vi "Modelo.vi"() -> ()   [LabVIEW 2016]
uses:
  <vilib>/addons/System Identification/Model Typedefs.llb/si_generic model.ctl
  <vilib>/addons/System Identification/Model Typedefs.llb/SI Model Type.ctl
  <vilib>/addons/System Identification/Model Typedefs.llb/si_variables.ctl
  <vilib>/addons/Control Design/_Model Construction/Model Typedefs.llb/CD Transfer Function Model (MIMO).ctl
  <vilib>/addons/Control Design/_Model Construction/Model Typedefs.llb/CD General Elements.ctl
  <vilib>/addons/Control Design/_Model Construction/Model Typedefs.llb/CD Transfer Function Model (SISO).ctl
  <vilib>/addons/Control Design/_PID Design/Datatypes/cd_PID Gains.ctl
  <vilib>/addons/Control Design/_PID Design/Datatypes/cd_Sampling Specifications.ctl
  <vilib>/Utility/file.llb/Read Delimited Spreadsheet (DBL).vi
  <vilib>/addons/Control Design/_Model Construction/Model Creation.llb/Model Creation SubVI/cd_Create Transfer Function Model.vi
  <vilib>/addons/Control Design/_PID Design/cd_Design PID for Discrete Systems (TF).vi
  <vilib>/Analysis/NI_AALPro.lvlib
  <vilib>/addons/Control Design/_PID Design/NI_CD_PID Design.lvlib
  <vilib>/addons/Control Design/_Model Construction/NI_LinSys_Model Creation.lvlib
  <vilib>/addons/System Identification/NI_SysID.lvlib
  <vilib>/addons/Control Design/_Model Construction/NI_LinSys_Model Typedefs.lvlib
panel:
  out "Design PID Gains":T1
  out "output cluster":T2 {"transfer function(s)"."delay" format="%.4f"; "transfer function(s)"."Denominator" format="%#_3g"; "transfer function(s)"."Numerator" format="%#_3g"; "properties"."Sampling Time" format="%#.6p"; "properties"."Output Delays" format="%.4f"; "properties"."Input Delays" format="%.4f"}
  out "size(s)":i32
  out "Waveform Graph":dbl[](graph)
  in  "file path (dialog if empty)":path
  out "coefficients":cluster{"numerator":dbl[], "denominator":dbl[]}
  out "system model out":T5={"attributes"={"version"="1.0", "model type"=0, "input names"=[], "output names"=[], "notes"=""}, "coefficients"={"A "=[], "B"=[], "F"=[], "C"=[], "D"=[]}, "std deviations"={"A "=[], "B"=[], "F"=[], "C"=[], "D"=[]}, "coefficients covariance"=[], "noise variance"=[], "fs"=0.0, "system info"={"number of inputs"=0, "number of outputs"=0, "A order"=[], "B order"=[], "F order"=[], "C order"=[], "D order"=[], "Delays"=[]}, "kalman gain"=[], "initial state"=[], "trans func"=[], "zeros-poles"=[], "std of trans func"=[], "std of zeros-poles"=[], "trans func (noise)"=[], "std of trans func (noise)"=[], "zeros-poles (noise)"=[], "std of zeros-poles (noise)"=[], "Symbolic State Space Model"={"Symbolic A"=[], "Symbolic B"=[], "Symbolic C"=[], "Symbolic D"=[], "Symbolic K"=[], "Symbolic Initial State"=[]}, "delay"=[], "variables"=[], "grey trans func spec"={"orders of TF model"={" num order"=1, "den order"=2}, "# of zeros/poles at origin"={"zeros/poles"=1, "number "=0}, "delay initial?"=FALSE, "gain initial?"=FALSE}} {"grey trans func spec"."# of zeros/poles at origin"."zeros/poles" items=["zeros", "poles"]; "std of zeros-poles (noise)"."gain" format="%.2f"; "std of zeros-poles (noise)"."poles" format="%.2f"; "std of zeros-poles (noise)"."zeros" format="%.2f"; "zeros-poles (noise)"."gain" format="%.2f"; "zeros-poles (noise)"."poles" format="%.2f"; "zeros-poles (noise)"."zeros" format="%.2f"; "std of trans func (noise)"."alphas" format="%.2f"; "std of trans func (noise)"."betas" format="%.2f"; "trans func (noise)"."alphas" format="%.2f"; "trans func (noise)"."betas" format="%.2f"; "std of zeros-poles"."gain" format="%.2f"; "std of zeros-poles"."poles" format="%.2f"; "std of zeros-poles"."zeros" format="%.2f"; "std of trans func"."alphas" format="%.2f"; "std of trans func"."betas" format="%.2f"; "zeros-poles"."gain" format="%.2f"; "zeros-poles"."poles" format="%.2f"; "zeros-poles"."zeros" format="%.2f"; "trans func"."alphas" format="%.2f"; "trans func"."betas" format="%.2f"; "fs" format="%.2f"; "std deviations"."A" format="%.2f"; "std deviations"."D" format="%.2f"; "std deviations"."C" format="%.2f"; "std deviations"."F" format="%.2f"; "std deviations"."B" format="%.2f"; "coefficients"."A" format="%.2f"; "coefficients"."D" format="%.2f"; "coefficients"."C" format="%.2f"; "coefficients"."F" format="%.2f"; "coefficients"."B" format="%.2f"; "attributes"."model type" items=["Undefined", "AR", "ARX (SISO)", "ARX (MISO)", "ARX (MIMO)", "ARMAX (SISO)", "ARMAX (MISO)", "Output-Error (SISO)", "Output-Error (MISO)", "Box-Jenkins (SISO)", "Box-Jenkins (MISO)", "General Linear (SISO)", "General Linear (MISO)", "State-Space (SISO)", "State-Space (MISO)", "State-Space (MIMO)", "Transfer Function (SISO)", "Transfer Function (MISO)", "Transfer Function (MIMO)", "Zero-Pole-Gain (SISO)", "Zero-Pole-Gain (MISO)", "Zero-Pole-Gain (MIMO)"]}
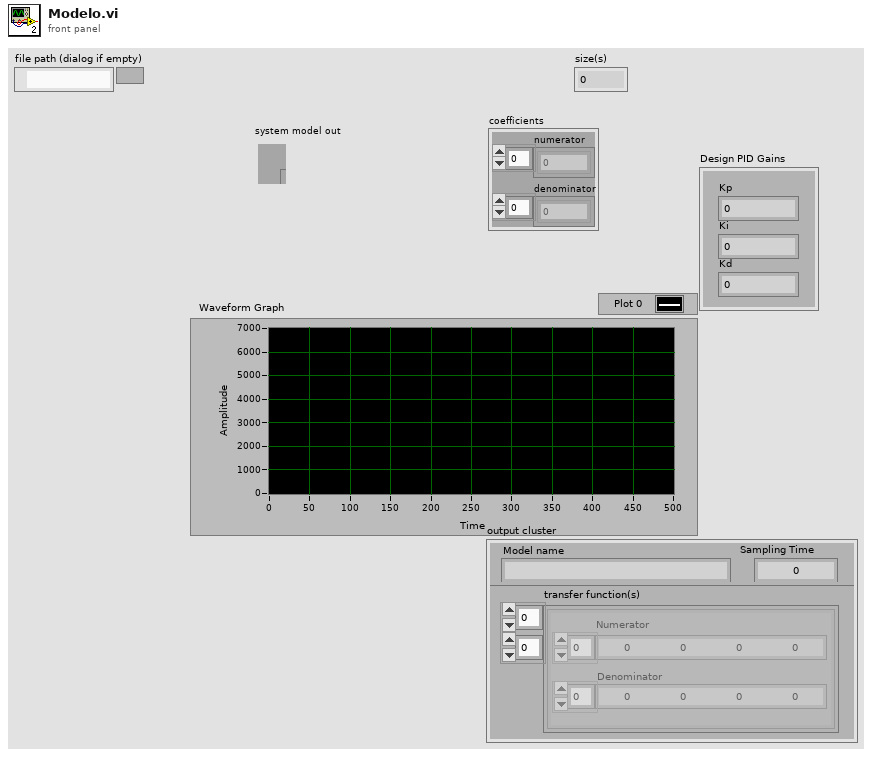
[diagram p1: front panel]
types:
  T1 = typedef "NI_CD_PID Design.lvlib/cd_PID Gains.ctl" = cluster{"Kp":dbl, "Ki":dbl, "Kd":dbl}
  T2 = typedef "NI_LinSys_Model Typedefs.lvlib/CD Transfer Function Model (MIMO).ctl" = cluster{"properties":T3, "transfer function(s)":T4[][]}
  T3 = typedef "NI_LinSys_Model Typedefs.lvlib/CD General Elements.ctl" = cluster{"Model name":string, "Input names":string[], "Output names":string[], "Input Delays":dbl[], "Output Delays":dbl[], "Sampling Time":dbl, "Notes":string}
  T4 = typedef "NI_LinSys_Model Typedefs.lvlib/CD Transfer Function Model (SISO).ctl" = cluster{"Numerator":dbl[], "Denominator":dbl[], "delay":dbl}
  T5 = typedef "NI_SysID.lvlib/si_generic model.ctl" = cluster{"attributes":cluster{"version":string, "model type":T6, "input names":string[], "output names":string[], "notes":string}, "coefficients":cluster{"A ":dbl[][][], "B":dbl[][][], "F":dbl[][][], "C":dbl[][][], "D":dbl[][][]}, "std deviations":cluster{"A ":dbl[][][], "B":dbl[][][], "F":dbl[][][], "C":dbl[][][], "D":dbl[][][]}, "coefficients covariance":dbl[][][], "noise variance":dbl[][], "fs":dbl, "system info":cluster{"number of inputs":i32, "number of outputs":i32, "A order":i32[][], "B order":i32[][], "F order":i32[][], "C order":i32[][], "D order":i32[][], "Delays":i32[][]}, "kalman gain":dbl[][], "initial state":dbl[], "trans func":cluster{"betas":dbl[], "alphas":dbl[]}[][], "zeros-poles":cluster{"zeros":cdb[], "poles":cdb[], "gain":dbl}[][], "std of trans func":cluster{"betas":dbl[], "alphas":dbl[]}[][], "std of zeros-poles":cluster{"zeros":cdb[], "poles":cdb[], "gain":dbl}[][], "trans func (noise)":cluster{"betas":dbl[], "alphas":dbl[]}[][], "std of trans func (noise)":cluster{"betas":dbl[], "alphas":dbl[]}[][], "zeros-poles (noise)":cluster{"zeros":cdb[], "poles":cdb[], "gain":dbl}[][], "std of zeros-poles (noise)":cluster{"zeros":cdb[], "poles":cdb[], "gain":dbl}[][], "Symbolic State Space Model":cluster{"Symbolic A":string[][], "Symbolic B":string[][], "Symbolic C":string[][], "Symbolic D":string[][], "Symbolic K":string[][], "Symbolic Initial State":string[]}, "delay":dbl[][], "variables":T7, "grey trans func spec":cluster{"orders of TF model":cluster{" num order":i32, "den order":i32}, "# of zeros/poles at origin":cluster{"zeros/poles":u16, "number ":i32}, "delay initial?":bool, "gain initial?":bool}}
  T6 = typedef "NI_SysID.lvlib/SI Model Type.ctl" = u16
  T7 = typedef "NI_SysID.lvlib/si_variables.ctl" = cluster{"name":string, "initial guess":dbl, "upper limit":dbl, "lower limit":dbl, "value":dbl}[]
  T8 = typedef "NI_CD_PID Design.lvlib/cd_Sampling Specifications.ctl" = cluster{"Num K Grid Points":u64, "Num Search Points":u64}
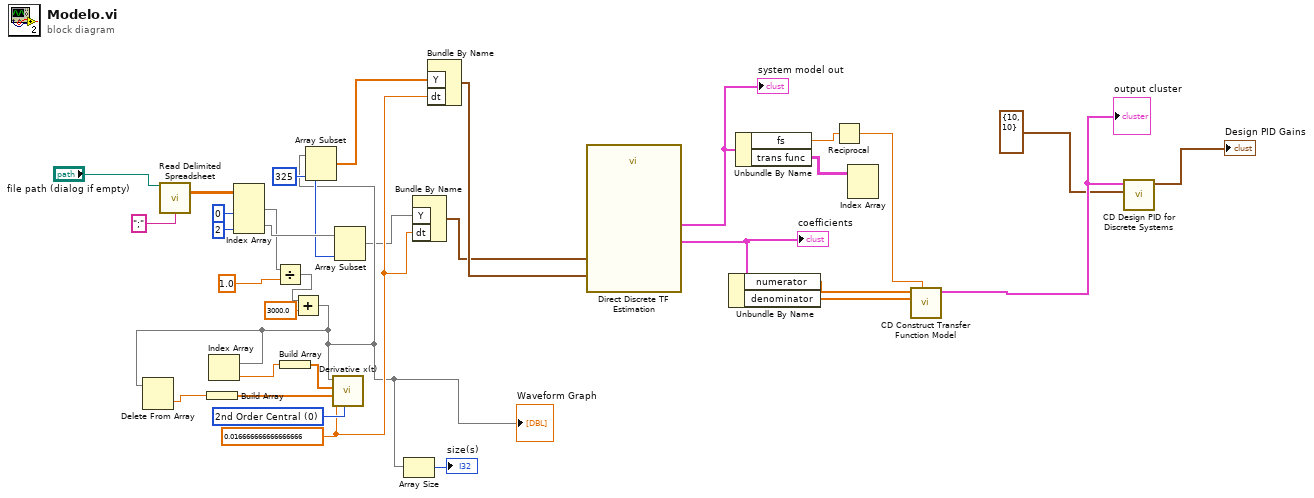
[diagram p0: block diagram]
diagram:
  w21 = 325 ("length")
  w18 = 0.016666666666666666 ("dt")
  w29 = u16 0 items=["2nd Order Central", "4th Order Central", "Forward", "Backward"] ("method")
  n1 = call-poly <vilib>:"Read Delimited Spreadsheet.vi"("file path (dialog if empty)"="file path (dialog if empty)", "delimiter (\\t)"=";" ("delimiter (\\t)")) -> ("all rows"=w23:dbl[][])  [unwired: 8 in, 5 out]
  n2 = Index Array(array=w23, index (col) #1=0 ("disabled index (col)"), index (col) #2=2 ("index (col)")) -> (element #1=w16:dbl[], element #2=w22:dbl[])  [unwired: 2 in]
  n3 = Divide(x=w16, y=1.0) -> (x/y=w6:dbl[])
  n4 = Add(x=w6, y=3000.0) -> (x+y=w4:dbl[])
  "Waveform Graph" <- w4
  n5 = Delete From Array(array=w4) -> (deleted portion=w26:dbl)  [unwired: 2 in, 1 out]
  n6 = Build Array(w26) -> (w25:dbl[])
  n7 = Index Array(array=w4) -> (element=w28:dbl)  [unwired: 1 in]
  n8 = Build Array(w28) -> (w27:dbl[])
  n9 = Array Subset(array=w4, length=w21) -> (w20:dbl[])  [unwired: 1 in]
  n10 = call <vilib>:"Derivative x(t).vi"("method"=w29, "dt"=w18, "Final Condition"=w25, "Initial Condition"=w27, "X"=w4) -> ()  [unwired: 5 in, 2 out]
  n11 = Array Subset(array=w22, length=w21) -> (w2:dbl[])  [unwired: 1 in]
  n12 = Array Size(array=w4) -> (size(s)=→"size(s)":i32)
  n13 = Bundle By Name("Y"=w2, "dt"=w18) -> (w17:waveform(dbl))  [unwired: 1 in]
  n14 = Bundle By Name("Y"=w20, "dt"=w18) -> (w19:waveform(dbl))  [unwired: 1 in]
  n15 = call "Direct Discrete TF Estimation"("response signal"=w19, "stimulus signal"=w17) -> ("coefficients"=w11:cluster{"numerator":dbl[], "denominator":dbl[]}, "system model out"=w14:T5)  [unwired: 7 in, 1 out]
  "system model out" <- w14
  "coefficients" <- w11
  n16 = Unbundle By Name(w11) -> ("numerator"=w10:dbl[], "denominator"=w9:dbl[])
  n17 = Unbundle By Name(w14) -> ("fs"=w12:dbl, "trans func"=w13:cluster{"betas":dbl[], "alphas":dbl[]}[][])
  n18 = Reciprocal(x=w12) -> (1/x=w8:dbl)
  n19 = Index Array(array=w13) -> ()  [unwired: 2 in, 1 out]
  n20 = call-poly <vilib>:"CD Construct Transfer Function Model.vi"("Sampling Time (s)"=w8, "Denominator"=w9, "Numerator"=w10) -> ("Transfer Function Model"=w3:T2)  [unwired: 7 in, 1 out]
  "output cluster" <- w3
  n21 = call-poly <vilib>:"CD Design PID for Discrete Systems.vi"("Sampling Specifications"=T8 {"Num K Grid Points"=10, "Num Search Points"=10}, "Transfer Function Model"=w3) -> ("Design PID Gains"=→"Design PID Gains":T1)  [unwired: 6 in, 3 out]
